vi "DefaultFromIni.vi"(8 "error in (no error)":errorcluster, 11 "SyncPlugin":refnum<class "NiPxi6682.lvclass">) -> (0 "error out":errorcluster, 3 "SyncPlugin":refnum<class "NiPxi6682.lvclass">)   [LabVIEW 2014, in "SyncPlugins.lvlib" / "NiPxi6682.lvclass"]
uses:
  NiPxi6682.lvclass
  Typedefs/clClkDest.ctl
  <userlib>/NIST/BaseClasses/BasePlugin_class/BasePlugin.lvclass/BasePlugin.ctl
  NiPxi6682.lvclass/NiPxi6682.ctl
  <userlib>/NIST/BaseClasses/BasePlugin_class/Accessors/Read PluginIniFilePath.vi
  Accessors/Write PgmPPS.vi
  Accessors/Write 1PPS.vi
  Accessors/Write DdsFreq.vi
  Accessors/Write PgmPPSFreq.vi
  Accessors/Write ClkDest.vi
  SyncPluginBase/SyncPluginBase.lvclass
  <vilib>/Utility/config.llb/NI_LVConfig.lvlib
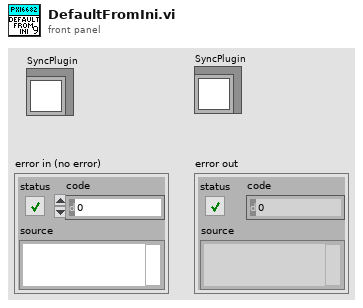
[diagram p1: front panel]
types:
  T1 = typedef "SyncPlugins.lvlib/NiPxi6682.lvclass/clClkDest.ctl" = cluster{"Term_1":string, "Term_2":string}
  T2 = typedef "NI_LVConfig.lvlib/Config Data RefNum.ctl" = refnum<k1>
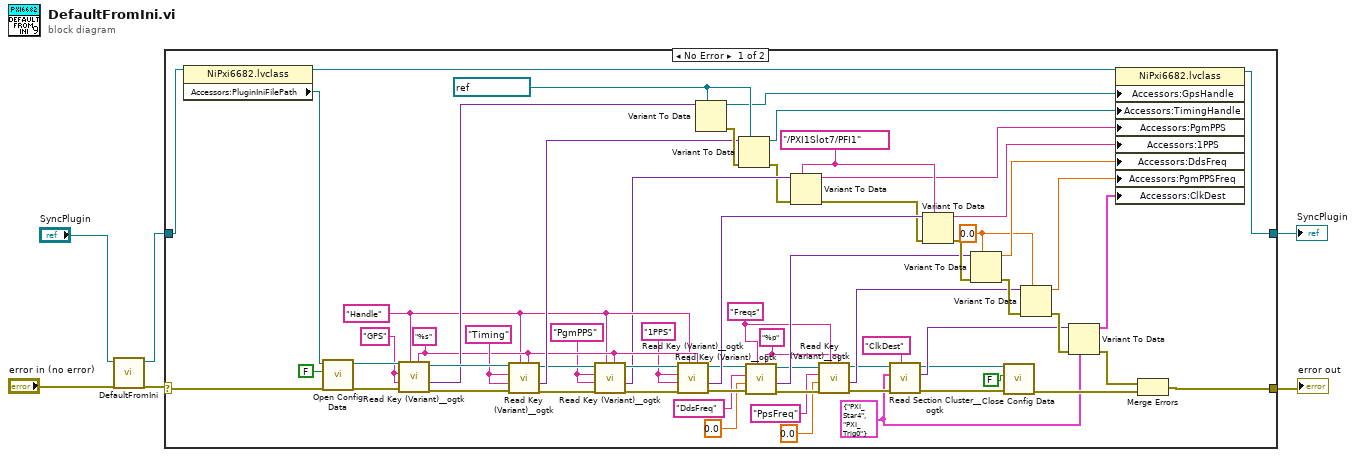
[diagram p0: block diagram]
diagram:
  n1 = call-parent "DefaultFromIni.vi"("error in (no error)"="error in (no error)", "SyncPlugin"="SyncPlugin") -> ("error out"=w4:errorcluster, "SyncPlugin"=w2:refnum<class "NiPxi6682.lvclass">)  [unwired: 8 in]
  n2 = case shown="No Error" w4 {
    selector: w4 -> [w66 w71]
    tunnel: [w35 w71] -> w3
    tunnel: [w55 w70] -> w1
    tunnel: w2 -> [w69 w70]
    frame No Error {
      w13 = T1 {"Term_1"="PXI_Star4", "Term_2"="PXI_Trig0"} ("ClkDest")
      w23 = "%p" ("format string (%;%f)")
      w24 = "Freqs" ("section")
      w19 = 0.0
      w37 = "1PPS" ("section")
      w38 = "PgmPPS" ("section")
      w41 = tag "/PXI1Slot7/PFI1" ("1PPS")
      w59 = refnum<k15> "PXI1Slot4" ("GpsHandle")
      w53 = "Timing" ("section")
      w47 = "%s" ("format string (%;%f)")
      w54 = "GPS" ("section")
      w46 = "Handle" ("section")
      n3 = property class="NiPxi6682.lvclass"(reference=w69) -> (reference out=w61:refnum<class "NiPxi6682.lvclass">, "Accessors:PluginIniFilePath"=w68:path)  [unwired: 1 in, 1 out]
      n4 = call <vilib>:"Open Config Data.vi"("error in (no error)"=w66, "create file if necessary (T)"=FALSE, "configuration file path"=w68) -> ("error out"=w65:errorcluster, "refnum"=w64:T2)  [unwired: 6 in, 1 out]
      n5 = call <userlib>:"Read Key (Variant)__ogtk.vi"("format string (%;%f)"=w47, "section"=w46, "error in (no error)"=w65, "type"=w54, "key (optional)"=w54, "refnum"=w64) -> ("error out"=w63:errorcluster, "key-value"=w60:variant, "refnum out"=w62:T2)  [unwired: 2 in, 1 out]
      n6 = call <userlib>:"Read Key (Variant)__ogtk.vi"("format string (%;%f)"=w47, "section"=w46, "error in (no error)"=w63, "type"=w53, "key (optional)"=w53, "refnum"=w62) -> ("error out"=w52:errorcluster, "key-value"=w51:variant, "refnum out"=w50:T2)  [unwired: 2 in, 1 out]
      n7 = call <userlib>:"Read Key (Variant)__ogtk.vi"("format string (%;%f)"=w47, "section"=w46, "error in (no error)"=w52, "type"=w38, "key (optional)"=w38, "refnum"=w50) -> ("error out"=w49:errorcluster, "key-value"=w45:variant, "refnum out"=w48:T2)  [unwired: 2 in, 1 out]
      n8 = call <userlib>:"Read Key (Variant)__ogtk.vi"("format string (%;%f)"=w47, "section"=w46, "error in (no error)"=w49, "type"=w37, "key (optional)"=w37, "refnum"=w48) -> ("error out"=w33:errorcluster, "key-value"=w44:variant, "refnum out"=w32:T2)  [unwired: 2 in, 1 out]
      n9 = Variant To Data(type=w59, Variant=w60) -> (data=w57:refnum<k15>, error out=w58:errorcluster)  [unwired: 1 in]
      n10 = Variant To Data(error in=w58, type=w59, Variant=w51) -> (data=w56:refnum<k15>, error out=w43:errorcluster)
      n11 = call <userlib>:"Read Key (Variant)__ogtk.vi"("format string (%;%f)"=w23, "section"=w24, "error in (no error)"=w33, "type"=0.0, "key (optional)"="DdsFreq", "refnum"=w32) -> ("error out"=w27:errorcluster, "key-value"=w26:variant, "refnum out"=w25:T2)  [unwired: 2 in, 1 out]
      n12 = Variant To Data(error in=w43, type=w41, Variant=w45) -> (data=w40:tag, error out=w42:errorcluster)
      n13 = call <userlib>:"Read Key (Variant)__ogtk.vi"("format string (%;%f)"=w23, "section"=w24, "error in (no error)"=w27, "type"=0.0, "key (optional)"="PpsFreq", "refnum"=w25) -> ("error out"=w17:errorcluster, "key-value"=w16:variant, "refnum out"=w15:T2)  [unwired: 2 in, 1 out]
      n14 = call <userlib>:"Read Section Cluster__ogtk.vi"("section (optional)"="ClkDest", "error in (no error)"=w17, "Section Formatted Cluster Type"=w13, "refnum"=w15) -> ("error out"=w9:errorcluster, "Section Formatted Cluster"=w11:variant, "dup refnum"=w10:T2)  [unwired: 3 in, 2 out]
      n15 = Variant To Data(error in=w42, type=w41, Variant=w44) -> (data=w39:tag, error out=w30:errorcluster)
      n16 = Variant To Data(error in=w30, type=w19, Variant=w26) -> (data=w31:dbl, error out=w20:errorcluster)
      n17 = call <vilib>:"Close Config Data.vi"("error in (no error)"=w9, "write file if changed (T)"=FALSE, "refnum"=w10) -> ("error out"=w36:errorcluster)  [unwired: 7 in, 1 out]
      n18 = Variant To Data(error in=w20, type=w19, Variant=w16) -> (data=w18:dbl, error out=w12:errorcluster)
      n19 = Variant To Data(error in=w12, type=w13, Variant=w11) -> (data=w7:T1, error out=w8:errorcluster)
      n20 = property class="NiPxi6682.lvclass"(reference=w61, "Accessors:GpsHandle"=w57, "Accessors:TimingHandle"=w56, "Accessors:PgmPPS"=w40, "Accessors:1PPS"=w39, "Accessors:DdsFreq"=w31, "Accessors:PgmPPSFreq"=w18, "Accessors:ClkDest"=w7) -> (reference out=w55:refnum<class "NiPxi6682.lvclass">)  [unwired: 1 in, 1 out]
      n21 = Merge Errors(w8, w36) -> (w35:errorcluster)
    }
    frame Error {
    }
  }
  "SyncPlugin" <- w1
  "error out" <- w3
